vi "Engine-UserPlugin.vi"(8 "Error In":errorcluster, 11 "DSI Reference":refnum<class "DCM-DSI.lvclass">) -> (0 "Error Out":errorcluster, 3 "DSI Reference":refnum<class "DCM-DSI.lvclass">)   [LabVIEW 2016, in "DSI-RT.lvlib"]
uses:
  DSI-RT.lvlib
  Classes/DCM-DSI/DCM-DSI.lvclass
  <vilib>/addons/Software Calibration Management/xSCM/CalPoint.xnode
  <vilib>/addons/Software Calibration Management/xSCM/FaultPoint.xnode
  <vilib>/addons/Software Calibration Management/xSCM/ni_scm.dll
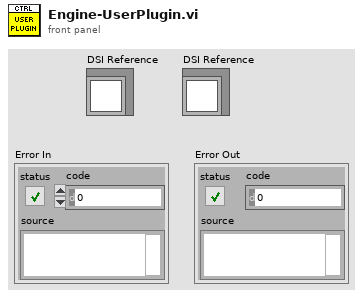
[diagram p1: front panel]
types:
  T1 = typedef "DSI-Shared.lvlib/UserParameter.ctl" = cluster{"Name":string, "Value":dbl}
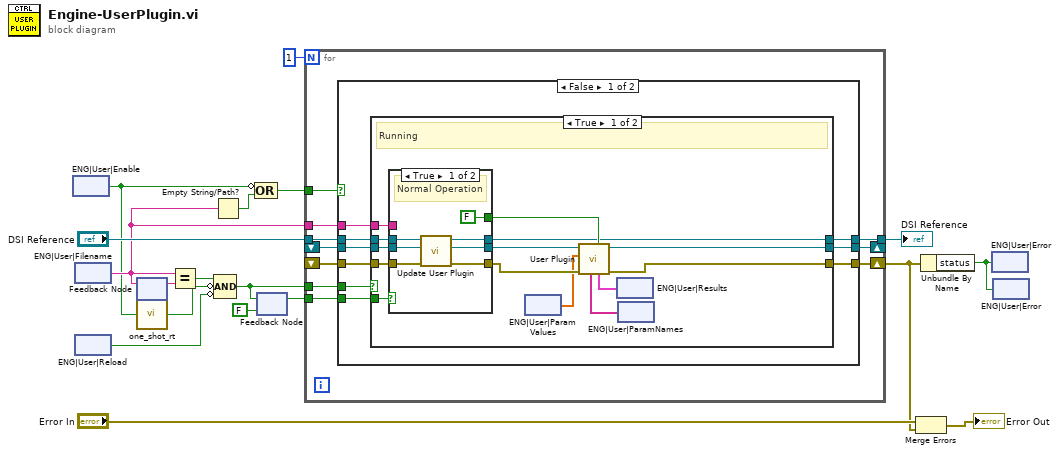
[diagram p0: block diagram]
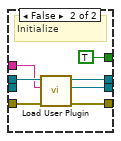
[diagram p2: hidden frame]
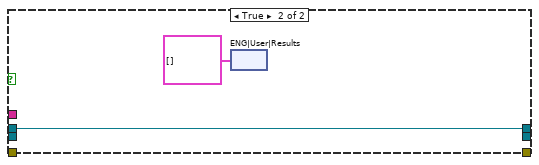
[diagram p4: hidden frame]
diagram:
  n1 = xnode "ENG|User|Enable"() -> ("Value"=w4:bool)
  n2 = xnode "ENG|User|Filename"() -> ("Value"=w10:string)
  n3 = xnode "ENG|User|Reload"() -> ("Value"=w3:bool)
  n4 = feedback #1() -> (w17:string)  [unwired: 1 in]
  n5 = feedback-in #1(w10) -> ()
  n6 = call <vilib>:"one_shot_rt.vi"("I"=w4) -> ("O"=w2:bool)
  n7 = Equal?(x=w10, y=w17) -> (x = y?=w15:bool)
  n8 = Empty String/Path?(string/path=w10) -> (empty?=w6:bool)
  n9 = Compound Arithmetic op=AND(w15, invert w2, invert w3) -> (w16:bool)
  n10 = Compound Arithmetic op=OR(invert w4, w6) -> (w5:bool)
  n11 = feedback #2(FALSE) -> (w18:bool)
  n12 = feedback-in #2(w16) -> ()
  n13 = for {
    N: 1 -> [_]
    tunnel: w18 -> [w28]
    tunnel: w16 -> [w27]
    tunnel: w10 -> [w26]
    tunnel: w5 -> [w25]
    shift-right: [w21] -> w8
    shift-left: _ -> [w23]
    tunnel: "DSI Reference" -> [w24]
    tunnel: [w22] -> w12
    shift-right: [w20] -> _
    shift-left: _ -> [w19]
    n14 = case shown="False" w25 {
      tunnel: [w37 w91] -> w22
      tunnel: [w36 _] -> w21
      tunnel: w28 -> [w35 _]
      tunnel: w27 -> [w34 _]
      tunnel: w26 -> [w33 _]
      tunnel: w24 -> [w32 w91]
      tunnel: w23 -> [w31 _]
      tunnel: [w30 _] -> w20
      tunnel: w19 -> [w29 _]
      frame False {
        n15 = case shown="True" w34 {
          tunnel: [w41 w89] -> w37
          tunnel: [w38 _] -> w36
          tunnel: w35 -> [w51 _]
          tunnel: w33 -> [w50 _]
          tunnel: w32 -> [w49 w89]
          tunnel: w31 -> [w48 _]
          tunnel: [w40 _] -> w30
          tunnel: w29 -> [w39 _]
          frame True {
            # "Running"
            n16 = case shown="True" w51 {
              tunnel: [w72 w80] -> w47
              tunnel: [w70 w81] -> w46
              tunnel: w50 -> [_ w77]
              tunnel: w49 -> [w75 w82]
              tunnel: w48 -> [w71 w78]
              tunnel: [FALSE ("Initialize") TRUE ("Initialize")] -> w42
              tunnel: [w73 w79] -> w41
              tunnel: w39 -> [w74 _]
              frame True {
                # "Normal Operation"
                n17 = call "Update User Plugin.vi"("error in (no error)"=w71, "Plugin Reference"=w74, "DSI Reference"=w75) -> ("error out"=w70:errorcluster, "Plugin Reference"=w72:refnum<class "DCM-DSI.lvclass">, "DSI Reference"=w73:refnum<class "DCM-DSI.lvclass">)  [unwired: 6 in]
              }
              frame False {
                # "Initialize"
                n18 = call "Load User Plugin.vi"("error in (no error)"=w78, "Name or relative path"=w77, "DSI Reference"=w82) -> ("error out"=w81:errorcluster, "Plugin Reference"=w80:refnum<class "DCM-DSI.lvclass">, "DSI Reference"=w79:refnum<class "DCM-DSI.lvclass">)  [unwired: 6 in]
              }
            }
            n19 = xnode "ENG|User|ParamValues"() -> ("Value"=w43:sgl[])
            n20 = call-dynamic "User Plugin.vi"("Initialize"=w42, "error in (no error)"=w46, "ParamValues"=w43, "DSI Reference"=w47) -> ("error out"=w38:errorcluster, "DSI Reference"=w40:refnum<class "DCM-DSI.lvclass">, "Results"=w44:T1[], "ParamNames"=w45:string[])  [unwired: 4 in]
            n21 = xnode "ENG|User|Results"("Value"=w44) -> ()
            n22 = xnode "ENG|User|ParamNames"("Value"=w45) -> ()
          }
          frame False {
            # "Off"
          }
        }
      }
      frame True {
        n23 = xnode "ENG|User|Results"("Value"=cluster{"Name":string, "Value":dbl}[] []) -> ()
      }
    }
  }
  "DSI Reference" <- w12
  n24 = Merge Errors("Error In", w8) -> (→"Error Out":errorcluster)
  n25 = Unbundle By Name(w8) -> ("status"=w7:bool)
  n26 = xnode "ENG|User|Error"("Value"=w7) -> ()
  n27 = xnode "ENG|User|Error"("Fault"=w7) -> ()
